vi "1D Array (Random[.0,1.]).vi"(1 "Length":u64=1, 4 "Scale(1.0)":dbl=1.0) -> (15 "Array":dbl[](array[numeric])=[0.8499685074535177, 0.8177846853127431, 0.14646651941963107, 0.9651673445548388, 0.9327823552328256, 0.5633081259489712] format="%_8f")   [LabVIEW 2014]
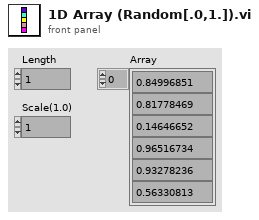
[diagram p1: front panel]
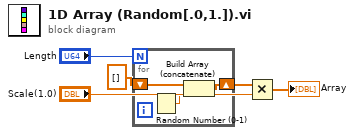
[diagram p0: block diagram]
diagram:
  n1 = for {
    N: "Length" -> [_]
    shift-right: [w7] -> w2
    shift-left: dbl[] [] -> [w6]
    n2 = Random Number (0-1)() -> (number: 0 to 1=w8:dbl)
    n3 = Build Array (concatenate)(w6, w8) -> (w7:dbl[])
  }
  n4 = Multiply(x=w2, y="Scale(1.0)") -> (x*y=→"Array":dbl[])
